vi "Save Data.vi"(4 "FileFormat":T9={"File Format"=enum."Macintosh (EOL: CR)", "Delimiter"=enum."TAB", "SaveComments?"=enum."Saved in the Header Area"}, 5 "Saving Mode":T1(ring), 6 "Data":dbl[](array[numeric]) format="%.2f", 8 "File Info Input":T3={"FilePath"=path "/DATA/Labview Items", "Field (T)"=55.0, "Temperature (K)"=77.0, "X-Axis"=enum."nm", "Center nm"=55.0, "Current Grating Density"=enum."600", "CCD Parameters"={"Exposure Time (s)"=0.2, "Offset"=0.0, "BkgrdCrct"=FALSE, "Shutter"=FALSE, "Mode"=enum."Regular", "Repetition"=4, "dt or s"=0.0}, "Operation Mode"=enum."NML Data Acquisition", "Exp Index"=0, "Index_repetition"=0, "Index"=0, "Current Detector"=enum."CCD-1024x256"} {"CCD Parameters"."dt or s" format="%#.6f"; "CCD Parameters"."Repetition" min=1; "CCD Parameters"."Offset" format="%#.2f"; "CCD Parameters"."Exposure Time (s)" min=0.02 max=6000.0 format="%#.2f"; "Center nm" format="%.2f"; "Temperature (K)" format="%.2f"; "Field (T)" format="%.2f"}, 9 "User Comments":string="This data's for you!\nType \u0011-H to get a help window for the various controls.", 10 "File Refnum":refnum<file>, 11 "File Parameter":T2={"Filename Prefix"="MyData", "Extension"=enum."±Field", "Suffix"="", "Current Path"=path "/opticsmac/Users/Data"}) -> (0 "File Info output":T3={"FilePath"=path "/DATA/Labview Items", "Field (T)"=55.0, "Temperature (K)"=77.0, "X-Axis"=enum."nm", "Center nm"=55.0, "Current Grating Density"=enum."600", "CCD Parameters"={"Exposure Time (s)"=0.2, "Offset"=0.0, "BkgrdCrct"=FALSE, "Shutter"=FALSE, "Mode"=enum."Regular", "Repetition"=4, "dt or s"=0.0}, "Operation Mode"=enum."NML Data Acquisition", "Exp Index"=0, "Index_repetition"=0, "Index"=0, "Current Detector"=enum."CCD-1024x256"} {"CCD Parameters"."dt or s" format="%#.6f"; "CCD Parameters"."Repetition" min=1; "CCD Parameters"."Offset" format="%#.2f"; "CCD Parameters"."Exposure Time (s)" min=0.02 max=6000.0 format="%#.2f"; "Center nm" format="%.2f"; "Temperature (K)" format="%.2f"; "Field (T)" format="%.2f"})   [LabVIEW 2020]
uses:
  Globals and TypeDefs/Type Definitions.llb/FileFormatParameter.ctt
  Globals and TypeDefs/Type Definitions.llb/FileInfoParameter.ctt
  Globals and TypeDefs/Type Definitions.llb/Wavelength Unit.ctt
  Globals and TypeDefs/Type Definitions.llb/McPherson Grating Density.ctl
  Globals and TypeDefs/Type Definitions.llb/CCDParameter.ctt
  Globals and TypeDefs/Type Definitions.llb/OperationMode.ctt
  Globals and TypeDefs/Type Definitions.llb/ListOfDetectors.ctt
  Globals and TypeDefs/Type Definitions.llb/FilePathParameter.ctt
  File and save/X-Axis Converter.llb/X-Axis Converter.vi
  File and save/X-Axis_Generator_morph.vi
panel:
  in  "error in":errorcluster
  out "Final File path":path
  out "Stop":bool=TRUE
  out "Contents Written":string
  out "Output File Name":string
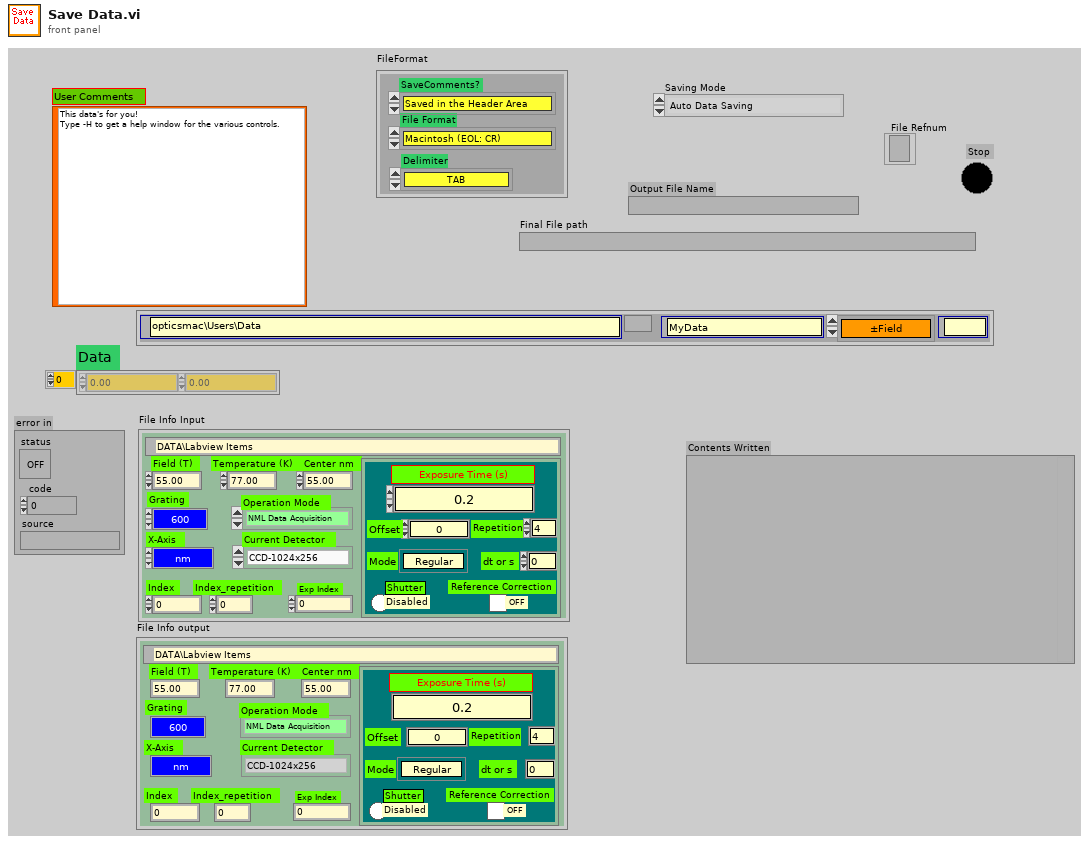
[diagram p1: front panel]
types:
  T1 = enum16{"Auto Data Saving", "Manual Data Saving", "Auto Sequence Saving", "Sequence Saving from Data Buffer"}
  T2 = typedef "FilePathParameter.ctt" = cluster{"Filename Prefix":string, "Extension":enum16{"none", "\".001\",\".002\", ...", "001 (No dot)", "±Field", "pField nField", "Temperature", "Wavelength", "T(K)±H(T)", "(nm)T(K)±H(T)", "User Defined"}, "Suffix":string, "Current Path":path}
  T3 = typedef "FileInfoParameter.ctt" = cluster{"FilePath":path, "Field (T)":dbl, "Temperature (K)":dbl, "X-Axis":T4, "Center nm":dbl, "Current Grating Density":T5, "CCD Parameters":T6, "Operation Mode":T7, "Exp Index":u32, "Index_repetition":u16, "Index":u16, "Current Detector":T8}
  T4 = typedef "Wavelength Unit.ctt" = enum8{"Point", "nm", "eV", "meV", "cm_1"}
  T5 = typedef "McPherson Grating Density.ctl" = enum8{"150", "300", "600", "1200", "1800"}
  T6 = typedef "CCDParameter.ctt" = cluster{"Exposure Time (s)":dbl, "Offset":dbl, "BkgrdCrct":bool, "Shutter":bool, "Mode":enum8{"Regular", "OverExp Cor", "SpikeRemove", "ForCalibration"}, "Repetition":u16, "dt or s":dbl}
  T7 = typedef "OperationMode.ctt" = enum16{"Standby", "CCD Single Shot", "CCD Sequence Shots", "CCD Custom Shots", "CCD Reference Shot", "Step Scanning ", "Time Scanning", "NML Data Acquisition"}
  T8 = typedef "ListOfDetectors.ctt" = enum8{"CCD-1024x256", "InGaAs PDA-1024x1", "CCD-1340x400", "Ge Single Channel", "Si Single Channel", "PMT Single Channel"}
  T9 = typedef "FileFormatParameter.ctt" = cluster{"File Format":enum16{"Macintosh (EOL: CR)", "Unix (EOL: LF)", "DOS/Windows (EOL: CR+LF)"}, "Delimiter":enum16{"TAB", "COMMA", "SPACE"}, "SaveComments?":enum16{"Bare data only", "Saved in the Header Area", "Saved as a Parameter File"}}
  T10 = enum16{"Bare data only", "Saved in the Header Area", "Saved as a Parameter File"}
  T11 = enum16{"Macintosh (EOL: CR)", "Unix (EOL: LF)", "DOS/Windows (EOL: CR+LF)"}
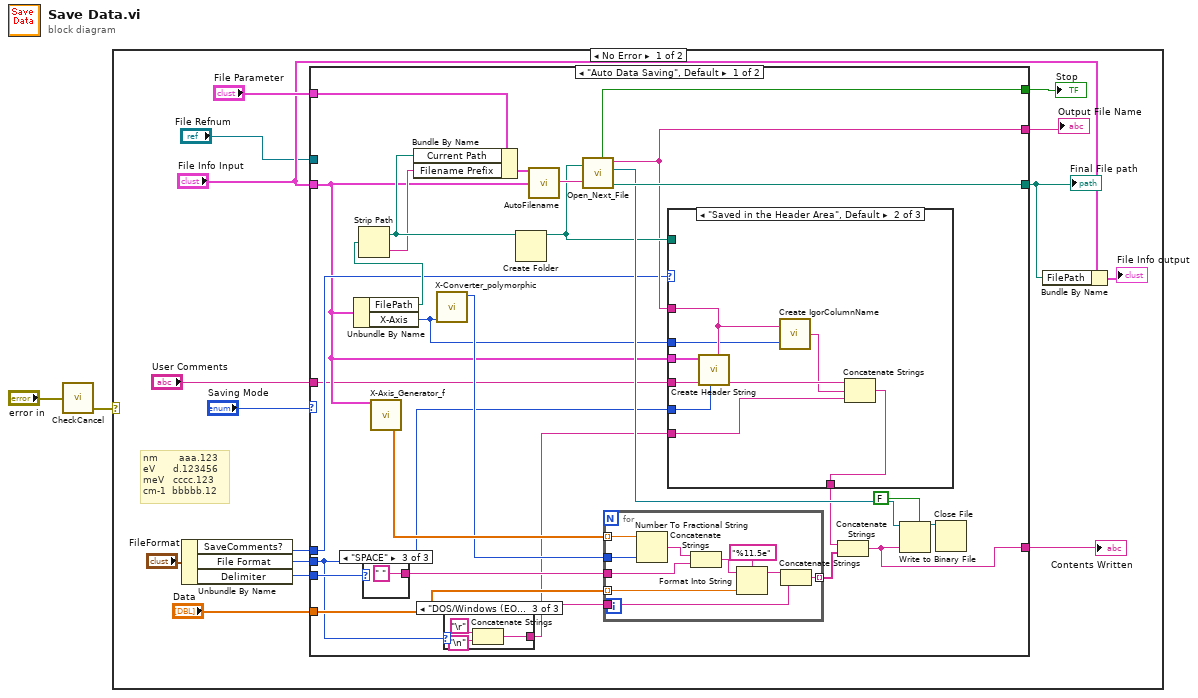
[diagram p0: block diagram]
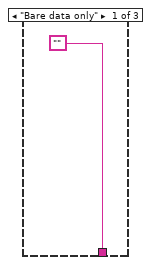
[diagram p2: hidden frame]
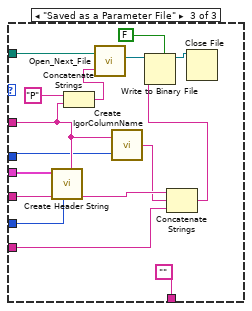
[diagram p3: hidden frame]
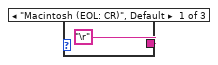
[diagram p4: hidden frame]
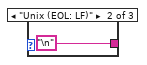
[diagram p5: hidden frame]
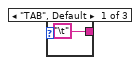
[diagram p6: hidden frame]
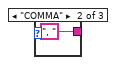
[diagram p7: hidden frame]
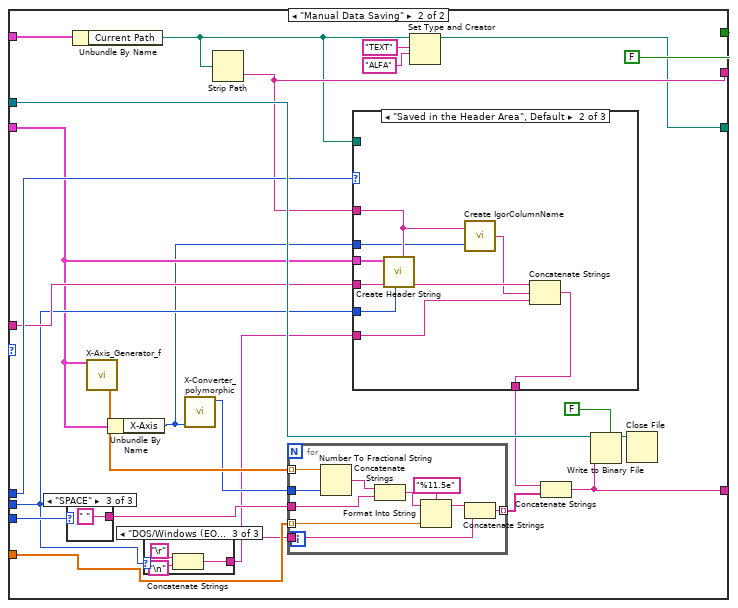
[diagram p8: hidden frame]
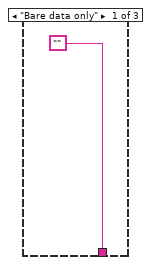
[diagram p9: hidden frame]
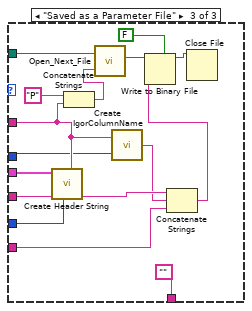
[diagram p10: hidden frame]
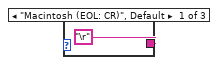
[diagram p11: hidden frame]
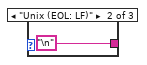
[diagram p12: hidden frame]
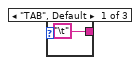
[diagram p13: hidden frame]
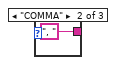
[diagram p14: hidden frame]
diagram:
  n1 = call "CheckCancel.vi"("error in (no error)"="error in") -> ("error out"=w1:errorcluster)  [unwired: 1 in, 1 out]
  n2 = case shown="No Error" w1 {
    frame No Error {
      # "nm       aaa.123\neV      d.123456\nmeV   cccc.123\ncm-1  bbbbb.12"
      n3 = Unbundle By Name("FileFormat") -> ("SaveComments?"=w10:T10, "File Format"=w12:T11, "Delimiter"=w11:enum16{"TAB", "COMMA", "SPACE"})
      n4 = case shown="\"Auto Data Saving\", Default" "Saving Mode" {
        tunnel: [w44 w91] -> w4
        tunnel: [w43 w111] -> w5
        tunnel: "User Comments" -> [w23 w97]
        tunnel: "File Parameter" -> [w31 w92]
        tunnel: "File Info Input" -> [w24 w94]
        tunnel: [w42 FALSE ("Stop")] -> w14
        tunnel: "Data" -> [w35 w104]
        tunnel: w12 -> [w22 w96]
        tunnel: w11 -> [w39 w107]
        tunnel: w10 -> [w25 w99]
        tunnel: [w26 w98] -> w9
        tunnel: "File Refnum" -> [_ w102]
        frame "Auto Data Saving", Default {
          n5 = Unbundle By Name(w24) -> ("FilePath"=w28:path, "X-Axis"=w20:T4)
          n6 = Strip Path(path=w28) -> (stripped path=w33:path, name=w32:string)
          n7 = case shown="\"SPACE\"" w39 {
            tunnel: ["\t" ", " " "] -> w40
            frame "TAB", Default {
            }
            frame "COMMA" {
            }
            frame "SPACE" {
            }
          }
          n8 = call-poly "X-Axis_Generator_f.vi"("File Info In"=w24) -> ("X-axis"=w36:dbl[])  [unwired: 11 in, 7 out]
          n9 = Bundle By Name(cluster=w31, "Current Path"=w33, "Filename Prefix"=w32) -> (w30:T2)
          n10 = call-poly "X-Converter_polymorphic.vi"("X-Axis Unit"=w20) -> ("Precision"=w34:i32)  [unwired: 4 in, 3 out]
          n11 = case shown="\"DOS/Windows (EOL: CR+LF)\"" w22 {
            tunnel: ["\r" "\n" w73] -> w21
            frame "Macintosh (EOL: CR)", Default {
            }
            frame "Unix (EOL: LF)" {
            }
            frame "DOS/Windows (EOL: CR+LF)" {
              n12 = Concatenate Strings("\r", "\n") -> (w73:string)
            }
          }
          n13 = Create Folder(path (use dialog)=w33) -> (created path=w27:path)  [unwired: 2 in, 2 out]
          n14 = call "AutoFilename.vi"("File Path Parameter"=w30, "File Info Parameter"=w24) -> ("FileNameOut"=w37:string)  [unwired: 11 in, 2 out]
          n15 = call "Open_Next_File.vi"("Input File Pattern"=w37, "Dir Path"=w27) -> ("Final File path"=w44:path, "File Ref Num"=w29:refnum<file>, "Output File Name"=w26:string, "Stop"=w42:bool)  [unwired: 1 out]
          n16 = for {
            tunnel: w35 -> [w83] mode=indexing
            tunnel: w36 -> [w86] mode=indexing
            tunnel: w34 -> [w87]
            tunnel: w40 -> [w85]
            tunnel: w21 -> [w80]
            tunnel: [w79] -> w38 mode=indexing
            n17 = Number To Fractional String(number=w86, precision (6)=w87) -> (F-format string=w88:string)  [unwired: 2 in]
            n18 = Concatenate Strings(w88, w85) -> (w84:string)
            n19 = Format Into String(format string="%11.5e", initial string=w84, w83) -> (resulting string=w81:string)  [unwired: 1 in, 1 out]
            n20 = Concatenate Strings(w81, w80) -> (w79:string)
          }
          n21 = case shown="\"Saved in the Header Area\", Default" w25 {
            tunnel: w26 -> [_ w49 w59]
            tunnel: w27 -> [_ _ w63]
            tunnel: w21 -> [_ w47 w57]
            tunnel: ["" w50 ""] -> w19
            tunnel: w24 -> [_ w54 w70]
            tunnel: w23 -> [_ w53 w69]
            tunnel: w22 -> [_ w52 w68]
            tunnel: w20 -> [_ w48 w58]
            frame "Bare data only" {
            }
            frame "Saved in the Header Area", Default {
              n22 = call "Create Header String.vi"("File Name"=w49, "File Format"=w52, "User Comments"=w53, "File Info Input"=w54) -> ("Contents Written"=w51:string)  [unwired: 7 in]
              n23 = call "Create IgorColumnName.vi"("X-Axis Unit"=w48, "FileName"=w49) -> ("Igor Column Names"=w46:string)
              n24 = Concatenate Strings(w51, w46, w47) -> (w50:string)
            }
            frame "Saved as a Parameter File" {
              n25 = call "Create Header String.vi"("File Name"=w59, "File Format"=w68, "User Comments"=w69, "File Info Input"=w70) -> ("Contents Written"=w67:string)  [unwired: 7 in]
              n26 = Concatenate Strings("P", w59) -> (w61:string)
              n27 = call "Open_Next_File.vi"("Input File Pattern"=w61, "Dir Path"=w63) -> ("File Ref Num"=w65:refnum<file>)  [unwired: 4 out]
              n28 = call "Create IgorColumnName.vi"("X-Axis Unit"=w58, "FileName"=w59) -> ("Igor Column Names"=w56:string)
              n29 = Concatenate Strings(w67, w56, w57) -> (w60:string)
              n30 = Write to Binary File(file (use dialog)=w65, data=w60, 5:FALSE ("prepend array or string size? (T)")) -> (refnum out=w64:refnum<file>)  [unwired: 3 in, 2 out]
              n31 = Close File(refnum=w64) -> ()  [unwired: 1 in, 2 out]
            }
          }
          n32 = Concatenate Strings(w19, w38) -> (w43:string)
          n33 = Write to Binary File(file (use dialog)=w29, data=w43, 5:FALSE ("prepend array or string size? (T)")) -> (refnum out=w41:refnum<file>)  [unwired: 3 in, 2 out]
          n34 = Close File(refnum=w41) -> ()  [unwired: 1 in, 2 out]
        }
        frame "Manual Data Saving" {
          n35 = case shown="\"SPACE\"" w107 {
            tunnel: ["\t" ", " " "] -> w108
            frame "TAB", Default {
            }
            frame "COMMA" {
            }
            frame "SPACE" {
            }
          }
          n36 = Unbundle By Name(w92) -> ("Current Path"=w91:path)
          n37 = call "X-Axis_Generator_f.vi"("File Info In"=w94) -> ("X-axis"=w105:dbl[])  [unwired: 11 in, 7 out]
          n38 = Unbundle By Name(w94) -> ("X-Axis"=w90:T4)
          n39 = case shown="\"DOS/Windows (EOL: CR+LF)\"" w96 {
            tunnel: ["\r" "\n" w140] -> w95
            frame "Macintosh (EOL: CR)", Default {
            }
            frame "Unix (EOL: LF)" {
            }
            frame "DOS/Windows (EOL: CR+LF)" {
              n40 = Concatenate Strings("\r", "\n") -> (w140:string)
            }
          }
          n41 = call-poly "X-Converter_polymorphic.vi"("X-Axis Unit"=w90) -> ("Precision"=w103:i32)  [unwired: 4 in, 3 out]
          n42 = Strip Path(path=w91) -> (name=w98:string)  [unwired: 1 out]
          n43 = for {
            tunnel: w104 -> [w150] mode=indexing
            tunnel: w105 -> [w153] mode=indexing
            tunnel: w103 -> [w154]
            tunnel: w108 -> [w152]
            tunnel: w95 -> [w147]
            tunnel: [w146] -> w106 mode=indexing
            n44 = Number To Fractional String(number=w153, precision (6)=w154) -> (F-format string=w155:string)  [unwired: 2 in]
            n45 = Concatenate Strings(w155, w152) -> (w151:string)
            n46 = Format Into String(format string="%11.5e", initial string=w151, w150) -> (resulting string=w148:string)  [unwired: 1 in, 1 out]
            n47 = Concatenate Strings(w148, w147) -> (w146:string)
          }
          n48 = case shown="\"Saved in the Header Area\", Default" w99 {
            tunnel: w98 -> [_ w116 w126]
            tunnel: w91 -> [_ _ w130]
            tunnel: w95 -> [_ w114 w124]
            tunnel: ["" w117 ""] -> w93
            tunnel: w94 -> [_ w121 w137]
            tunnel: w97 -> [_ w120 w136]
            tunnel: w96 -> [_ w119 w135]
            tunnel: w90 -> [_ w115 w125]
            frame "Bare data only" {
            }
            frame "Saved in the Header Area", Default {
              n49 = call "Create Header String.vi"("File Name"=w116, "File Format"=w119, "User Comments"=w120, "File Info Input"=w121) -> ("Contents Written"=w118:string)  [unwired: 7 in]
              n50 = call "Create IgorColumnName.vi"("X-Axis Unit"=w115, "FileName"=w116) -> ("Igor Column Names"=w113:string)
              n51 = Concatenate Strings(w118, w113, w114) -> (w117:string)
            }
            frame "Saved as a Parameter File" {
              n52 = call "Create Header String.vi"("File Name"=w126, "File Format"=w135, "User Comments"=w136, "File Info Input"=w137) -> ("Contents Written"=w134:string)  [unwired: 7 in]
              n53 = Concatenate Strings("P", w126) -> (w128:string)
              n54 = call "Open_Next_File.vi"("Input File Pattern"=w128, "Dir Path"=w130) -> ("File Ref Num"=w132:refnum<file>)  [unwired: 4 out]
              n55 = call "Create IgorColumnName.vi"("X-Axis Unit"=w125, "FileName"=w126) -> ("Igor Column Names"=w123:string)
              n56 = Concatenate Strings(w134, w123, w124) -> (w127:string)
              n57 = Write to Binary File(file (use dialog)=w132, data=w127, 5:FALSE ("prepend array or string size? (T)")) -> (refnum out=w131:refnum<file>)  [unwired: 3 in, 2 out]
              n58 = Close File(refnum=w131) -> ()  [unwired: 1 in, 2 out]
            }
          }
          n59 = Set Type and Creator(5:"ALFA", 6:"TEXT", 7:w91) -> ()  [unwired: 1 in, 2 out]
          n60 = Concatenate Strings(w93, w106) -> (w111:string)
          n61 = Write to Binary File(file (use dialog)=w102, data=w111, 5:FALSE ("prepend array or string size? (T)")) -> (refnum out=w109:refnum<file>)  [unwired: 3 in, 2 out]
          n62 = Close File(refnum=w109) -> ()  [unwired: 1 in, 2 out]
        }
      }
      "Contents Written" <- w5
      "Stop" <- w14
      "Output File Name" <- w9
      "Final File path" <- w4
      n63 = Bundle By Name(cluster="File Info Input", "FilePath"=w4) -> (→"File Info output":T3)
    }
    frame Error {
    }
  }
